vi "Read DAQ FIFO.vi"(8 "error in (no error)":errorcluster, 9 "Timeout (ms)":i32, 10 "Data In":T1[](array[typedef]), 11 "CIF_NIChn_FIFO_DAQ in":refnum<class "CIF_NIChn_FIFO_DAQ.lvclass">) -> (0 "error out":errorcluster, 1 "timed out?":bool, 2 "Data Out":T1[](array[typedef]), 3 "CIF_NIChn_FIFO_DAQ out":refnum<class "CIF_NIChn_FIFO_DAQ.lvclass">, 4 "Header":T2)   [LabVIEW 2021, in "CIF_NIChn_FIFO_DAQ.lvclass"]
uses:
  CIF_NIChn_FIFO_DAQ.lvclass
  D:/dev/Packages/Channel_Manager/src/CIF_NIChn/NIChn/CIF_NIChn.lvclass
  D:/dev/Packages/Channel_Manager/src/CIFChannels/CIFChannels.lvclass
  ChannelCommon/typedef/FIFO Header.ctl
  ChannelCommon/typedef/Datatype Waveform.ctl
  NIChn/CIF_NIChn.lvclass/CIF_NIChn.ctl
  CIFChannels/CIFChannels.lvclass/CIFChannels.ctl
  <vilib>/CIF Foundation/CIF Utilities/Statistics/I64/Stats_I64_CIF_U.lvclass/Stats_I64_CIF_U.ctl
  NIChn/Accessors/Read CIF Channel.vi
  ChannelCommon/Utilities/Unflatten Header.vi
  <vilib>/CIF Foundation/CIF Utilities/DataTypes/Unflatten I64.vi
  <vilib>/CIF Foundation/CIF Utilities/DataTypes/Unflatten U64.vi
  <vilib>/CIF Foundation/CIF Channels/CIFChannels/Top Level/Read U8 Array.vi
  <vilib>/CIF Foundation/CIF Channels/CIFChannels/Top Level/Advanced/Read U8 FIFO as Dbl Array.vi
  CIFChannels/Utilities/Update Channel Benchmark.vi
  SubVIs/Read and Unflatten.vi/8d434fcd-ba02-44c6-a1d2-d54d1c5f4ff9.vi
  SubVIs/Read and Unflatten.vi/c632fbd8-b242-46ac-b145-31e81b296fef.vi
  ChannelCommon/Utilities/Add Error.vi
  <vilib>/CIF Foundation/CIF Channels/CIFChannels/Top Level/Read U8 Array.vi/4bc1c15b-36ab-481f-b8dd-c64075ce723a.vi
  <vilib>/CIF Foundation/CIF Channels/CIFChannels/Top Level/Read U8 Array.vi/d83cb72b-7713-41fc-a3d1-682de79cf574.vi
  <vilib>/CIF Foundation/CIF Channels/CIFChannels/SubVIs/Get dll Path.vi
  <vilib>/CIF Foundation/CIF Channels/CIFChannels/SubVIs/Get Requested Size.vi
  <vilib>/CIF Foundation/CIF Channels/CIFChannels/Top Level/Advanced/Read U8 FIFO as Dbl Array.vi/4bc1c15b-36ab-481f-b8dd-c64075ce723a.vi
  <vilib>/CIF Foundation/CIF Channels/CIFChannels/Top Level/Advanced/Read U8 FIFO as Dbl Array.vi/d83cb72b-7713-41fc-a3d1-682de79cf574.vi
  <vilib>/CIF Foundation/CIF Utilities/Statistics/I64/X1 minus X0.vi
  <vilib>/CIF Foundation/CIF Utilities/Time/System Time/Get System Time.vi
  <vilib>/CIF Foundation/CIF Utilities/Errors/Append Error Location.vi
  <vilib>/CIF Foundation/CIF Utilities/Statistics/I64/X1 minus X0.vi/dfabcf33-0dbc-4041-80a5-3dc0c86d2989.vi
  <vilib>/CIF Foundation/CIF Utilities/Time/System Time/LabVIEW Time to TAI Time.vi
  <vilib>/CIF Foundation/CIF Utilities/Statistics/I64/X1 minus X0.vi/dfabcf33-0dbc-4041-80a5-3dc0c86d2989.vi/9eb60a9a-770f-4d2d-8b3f-8465c267ecc9.vi
  CIF_NIChn_FIFO_DAQ.lvclass/CIF_NIChn_FIFO_DAQ.ctl
  FIFO_U8/CIF_NIChn_Fifo_U8.lvclass
  D:/dev/Packages/Channel_Manager/src/CIF_NIChn/FIFO_U8/CIF_NIChn_Fifo_U8.lvclass
  ChannelCommon/ChannelCommon.lvlib
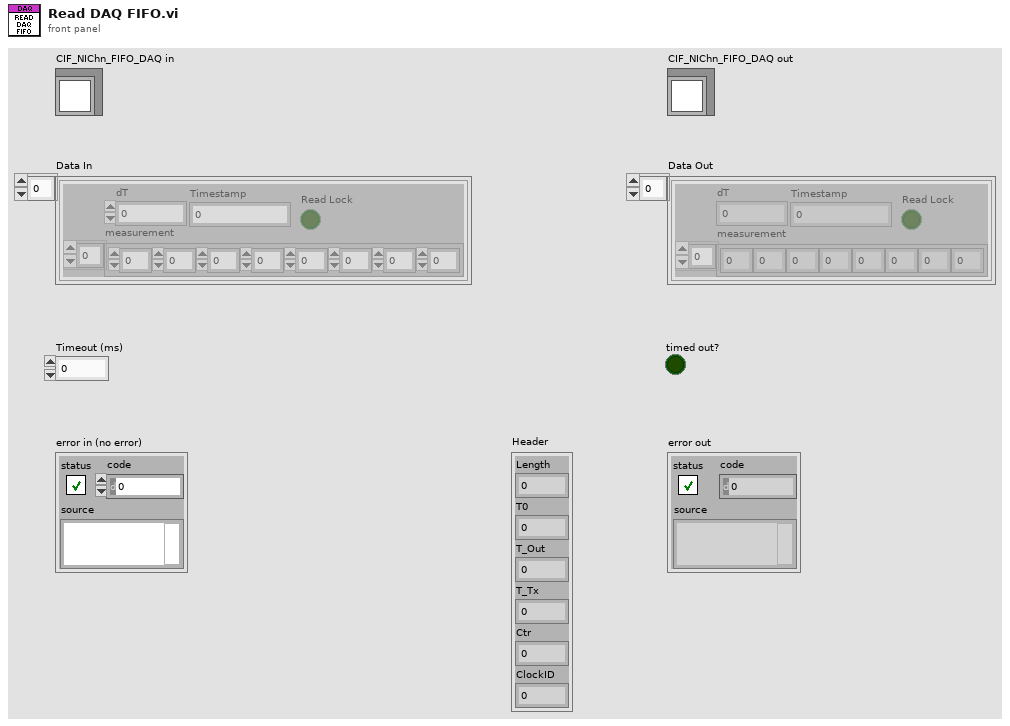
[diagram p1: front panel]
types:
  T1 = typedef "ChannelCommon.lvlib/Datatype Waveform.ctl" = cluster{"measurement":dbl[], "dT":dbl, "Timestamp":i64, "Read Lock":bool}
  T2 = typedef "ChannelCommon.lvlib/FIFO Header.ctl" = cluster{"Length":u64, "T0":i64, "T_Out":i64, "T_Tx":i64, "Ctr":u64, "ClockID":u8}
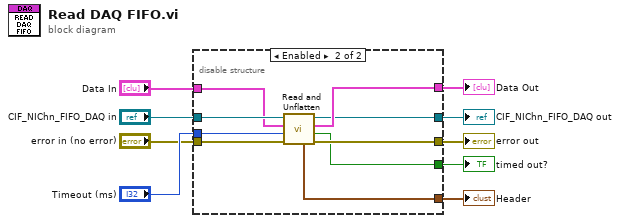
[diagram p0: block diagram]
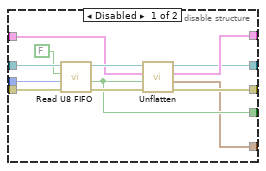
[diagram p2: hidden frame]
diagram:
  n1 = disable-structure shown="Enabled" {
    disable-tunnel: "CIF_NIChn_FIFO_DAQ in" -> [w21 w29]
    disable-tunnel: "Timeout (ms)" -> [w20 w22]
    disable-tunnel: "error in (no error)" -> [w19 w30]
    disable-tunnel: "Data In" -> [w15 w28]
    disable-tunnel: [w14 w24] -> w5
    disable-tunnel: [w13 w27] -> w4
    disable-tunnel: [w12 w26] -> w3
    disable-tunnel: [w11 w25] -> w2
    disable-tunnel: [w10 w23] -> w1
    frame Disabled {
      n2 = call "Read U8 FIFO.vi"("error in (no error)"=w19, "Timeout (ms)"=w20, "Return Data"=FALSE, "CIFFIFO in"=w21) -> ("error out"=w16:errorcluster, "timed out?"=w14:bool, "CIFFIFO out"=w18:refnum<class "CIF_NIChn_FIFO_DAQ.lvclass">)  [unwired: 3 in, 2 out]
      n3 = call "Unflatten.vi"("error in (no error)"=w16, "Timeout"=w14, "DAQ In"=w15, "CIF_NIChn_FIFO_DAQ in"=w18) -> ("error out"=w11:errorcluster, "Header"=w10:T2, "DAQ Out"=w13:T1[], "CIF_NIChn_FIFO_DAQ out"=w12:refnum<class "CIF_NIChn_FIFO_DAQ.lvclass">)  [unwired: 4 in]
    }
    frame Enabled {
      n4 = call "Read and Unflatten.vi"("error in (no error)"=w30, "Timeout (ms)"=w22, "Data in"=w28, "CIF_NIChn_FIFO_DAQ in"=w29) -> ("error out"=w25:errorcluster, "Timed out?"=w24:bool, "Data out"=w27:T1[], "CIF_NIChn_FIFO_DAQ out"=w26:refnum<class "CIF_NIChn_FIFO_DAQ.lvclass">, "Header out"=w23:T2)  [unwired: 3 in]
    }
  }
  "error out" <- w2
  "CIF_NIChn_FIFO_DAQ out" <- w3
  "timed out?" <- w5
  "Header" <- w1
  "Data Out" <- w4
